vi "VersaoCuppoGerador.vi"() -> ()   [LabVIEW 2018]
uses:
  <vilib>/measure/maspectr.llb/FFT Power Spectrum and PSD for 1 Chan.vi
  <vilib>/express/express analysis/Spectral/Block/exnSpectralBlock spectral measurements peak poly.vi
  <vilib>/express/express analysis/Spectral/Block/exnSpectralBlock spectral measurements peak WFM.vi
  <vilib>/express/express analysis/Spectral/XNode/ExpressSpectralMeasurementsBlockNode.xnode
  <vilib>/Analysis/NI_AALPro.lvlib
  <vilib>/measure/NI_MAPro.lvlib
panel:
  out "Power Spectrum / PSD":cluster{"f0":dbl, "df":dbl, "magnitude":dbl[]} {"magnitude" format="%.2p"; "f0" format="%0.2p"; "df" format="%0.2p"}
  out "XY Graph 3":cluster{dbl[], dbl[]}(graph)
  out "Waveform Graph":cluster{"f0":dbl, "df":dbl, "magnitude":dbl[]}(graph)
  out "XY Graph 2":cluster{dbl[], dbl[]}(graph)
  out "XY Graph":cluster{dbl[], dbl[]}(graph)
  in  "stop":bool
  in  "Número de Harmônicas":dbl=4.0
  in  "Amplitude":dbl=2.0
  in  "Frequência":dbl=10.0
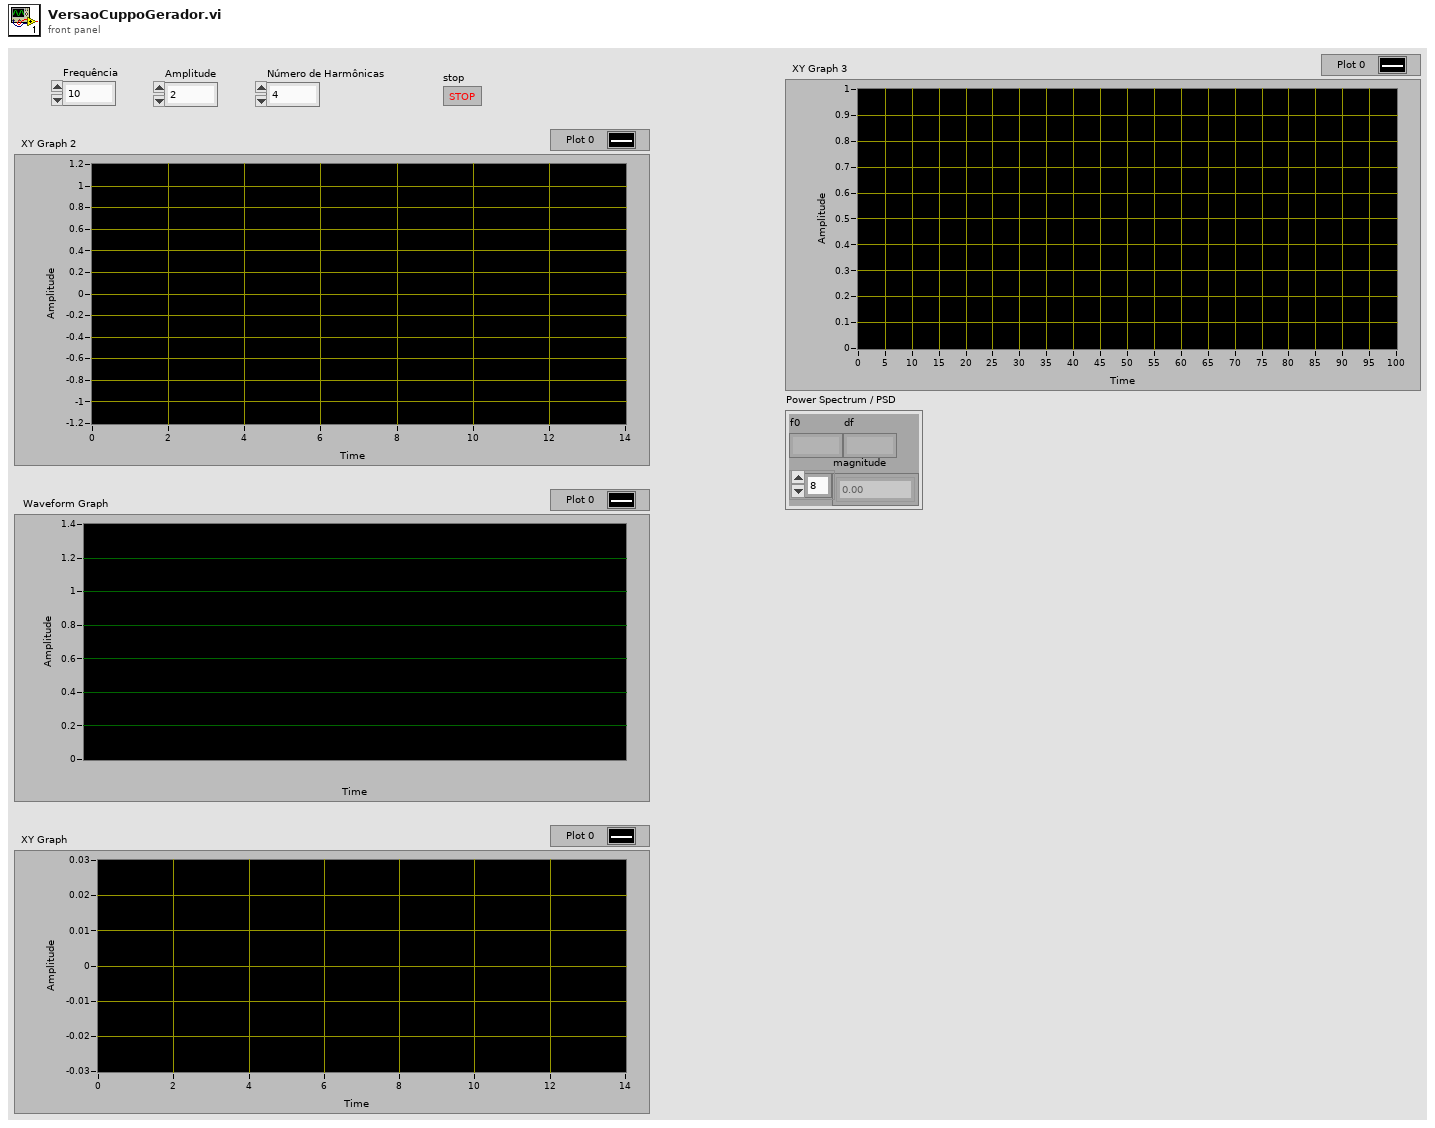
[diagram p1: front panel]
types:
  T1 = cluster{"averaging mode":u16, "weighting mode":u16, "number of averages":u32}
  T2 = cluster{"dB On (F)":bool, "unwrap phase (F)":bool, "convert to degree (F)":bool}
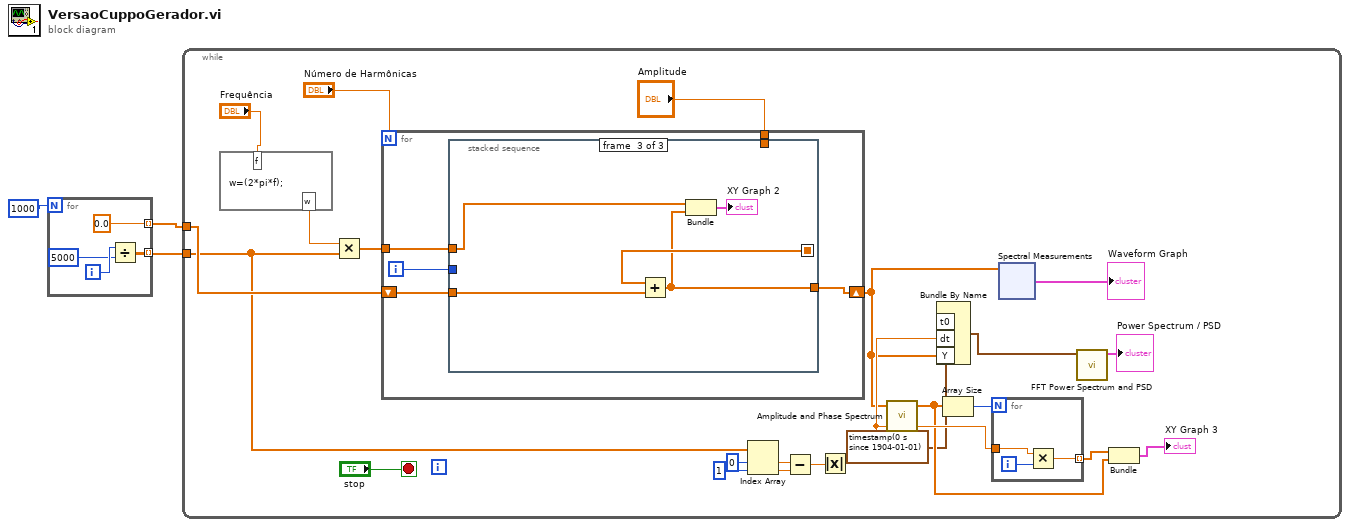
[diagram p0: block diagram]
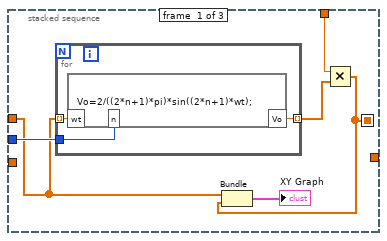
[diagram p2: hidden frame]
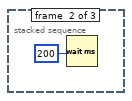
[diagram p3: hidden frame]
diagram:
  n1 = for {
    N: 1000 -> [_]
    tunnel: [w5] -> w2 mode=indexing
    tunnel: [0.0 ("Frequência 2")] -> w1 mode=indexing
    i -> [w7]
    n2 = Divide(x=w7, y=5000) -> (x/y=w5:dbl)
  }
  n3 = while {
    tunnel: w2 -> [w24]
    tunnel: w1 -> [w26]
    stop <- "stop" stop-if-true
    n4 = formula code="w=(2*pi*f);"("f"="Frequência") -> ("w"=w28:dbl)
    n5 = Multiply(x=w28, y=w24) -> (x*y=w29:dbl[])
    n6 = for {
      N: "Número de Harmônicas" -> [_]
      tunnel: w29 -> [w48]
      shift-right: [w46] -> w12
      shift-left: w26 -> [w47]
      tunnel: "Amplitude" -> [w45]
      i -> [w49]
      n7 = stacked-sequence {
        seq-local: [w50 _ _] -> [_ _ w63]
        tunnel: w49 -> [w55 _ _]
        tunnel: w48 -> [w53 _ w62]
        tunnel: w47 -> [_ _ w64]
        tunnel: [_ _ w61] -> w46
        tunnel: w45 -> [w52 _ _]
        frame #0 {
          n8 = for {
            tunnel: w53 -> [w58] mode=indexing
            tunnel: w55 -> [w57]
            tunnel: [w56] -> w51 mode=indexing
            n9 = formula code="Vo=2/((2*n+1)*pi)*sin((2*n+1)*wt);"("wt"=w58, "n"=w57) -> ("Vo"=w56:dbl)
          }
          n10 = Multiply(x=w52, y=w51) -> (x*y=w50:dbl[])
          n11 = Bundle(w53, w50) -> (→"XY Graph":cluster{dbl[], dbl[]})  [unwired: 1 in]
        }
        frame #1 {
          n12 = Wait (ms)(milliseconds to wait=200) -> ()  [unwired: 1 out]
        }
        frame #2 {
          n13 = Add(x=w63, y=w64) -> (x+y=w61:dbl[])
          n14 = Bundle(w62, w61) -> (→"XY Graph 2":cluster{dbl[], dbl[]})  [unwired: 1 in]
        }
      }
    }
    n15 = Index Array(array=w24, index #1=0 ("index"), index #2=1 ("index")) -> (element #1=w21:dbl, element #2=w20:dbl)
    n16 = Subtract(x=w21, y=w20) -> (x-y=w19:dbl)
    n17 = Absolute Value(x=w19) -> (abs(x)=w13:dbl)
    n18 = call <vilib>:"Amplitude and Phase Spectrum.vi"("dt"=w13, "Signal (V)"=w12) -> ("df"=w17:dbl, "Amp Spectrum Mag (Vrms)"=w14:dbl[])  [unwired: 1 in, 1 out]
    n19 = Bundle By Name("t0"=timestamp(0 s since 1904-01-01), "dt"=w13, "Y"=w12) -> (w10:waveform(dbl))  [unwired: 1 in]
    n20 = Array Size(array=w14) -> (size(s)=w18:i32)
    n21 = for {
      N: w18 -> [_]
      tunnel: w17 -> [w33]
      tunnel: [w32] -> w16 mode=indexing
      i -> [w34]
      n22 = Multiply(x=w33, y=w34) -> (x*y=w32:dbl)
    }
    n23 = xnode "Spectral Measurements"("Signals"=w12) -> ("FFT - (Peak)"=→"Waveform Graph":cluster{"f0":dbl, "df":dbl, "magnitude":dbl[]})  [unwired: 1 in, 2 out]
    n24 = call-poly <vilib>:"FFT Power Spectrum and PSD.vi"("time signal"=w10) -> ("Power Spectrum / PSD"=→"Power Spectrum / PSD":cluster{"f0":dbl, "df":dbl, "magnitude":dbl[]})  [unwired: 7 in, 3 out]
    n25 = Bundle(w16, "Amp Spectrum Mag (Vrms)"=w14) -> (→"XY Graph 3":cluster{dbl[], "Amp Spectrum Mag (Vrms)":dbl[]})  [unwired: 1 in]
  }
